vi "ZMC Make Real Zpj Mem.vi"(8 "error in (no error)":errorcluster caption="错误输入（无错误）", 10 "pzpj":u32, 11 "pBasDir":string) -> (0 "error out":errorcluster caption="错误输出", 2 "pzpj out":u32, 3 "function return":i32)   [LabVIEW 2015, in "zauxdll.lvlib"]
doc: "int32 __stdcall ZMC_MakeRealZpjMem(const char* pBasDir, void *pzpj);"
uses:
  zauxdll.lvlib
  zmotion.dll
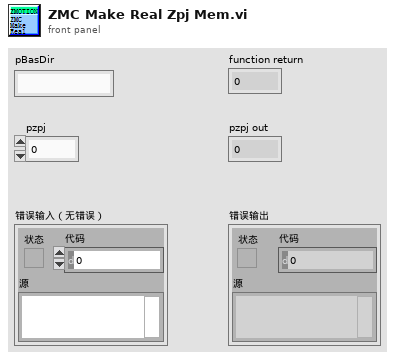
[diagram p1: front panel]
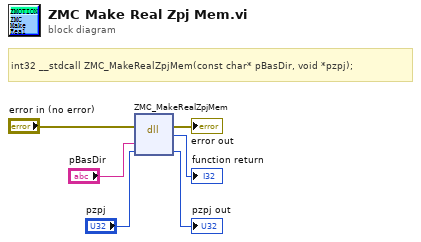
[diagram p0: block diagram]
diagram:
  # "int32 __stdcall ZMC_MakeRealZpjMem(const char* pBasDir, void *pzpj);"
  n1 = dll-call lib="C:/Users/VIC/Desktop/GOGORO_SA/system/LLB/zmotion/zaux/zmotion.*" fn="ZMC_MakeRealZpjMem"(error in="error in (no error)", "pBasDir"="pBasDir", "pzpj"="pzpj") -> (error out=→"error out":errorcluster, →"function return":i32, "pzpj"=→"pzpj out":u32)  [unwired: 3 in, 1 out]
